vi "Fetch Measurement (Others).vi"(0 "VISA resource name":refnum<visa-resource-name>, 5 "Timeout (10000 ms)":i32=10000 format="%.0g", 7 "Fetch Option (0)":i32, 11 "error in (no error)":errorcluster) -> (4 "VISA resource name out":refnum<visa-resource-name>, 6 "Measurement Data":dbl[](array[numeric]), 15 "error out":errorcluster)   [LabVIEW 2014, in "Agilent MXA Series.lvlib"]
doc: "Returns the results of last measurement(ACP, Burst Power, Spurious Emissions, Spectrum Emission Mask) and does not initiate data acquisition.\n\n<B>Note:</B>\n\nUse this VI only with other low-level VIs. The high-level VIs automatically incorporate this functionality. This VI does not check the instrument status."
uses:
  Agilent MXA Series.lvlib
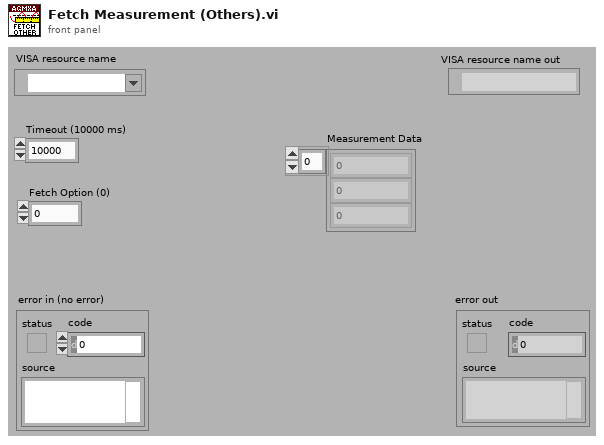
[diagram p1: front panel]
types:
  T1 = typedef "Agilent MXA Series.lvlib/Extended User Data.ctl" = cluster{"Measurement Type":i32, "Agilent MXA/EXA Model":i32}
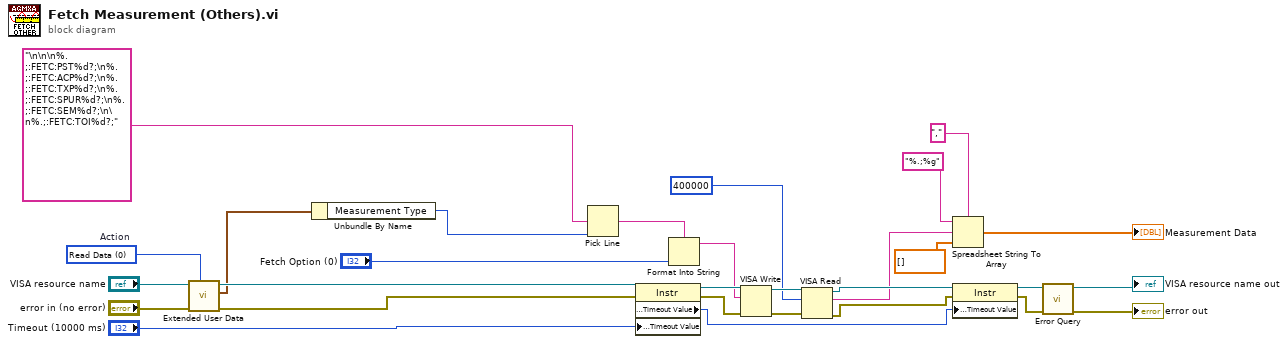
[diagram p0: block diagram]
diagram:
  w10 = 0 items=["Read Data", "Write Data", "Clear Data", "Clear ALL Data"]  # Action
  n1 = call "Extended User Data.vi"("Action (1:Write Data)"=w10, "Error In (no error)"="error in (no error)", "VISA resource name in"="VISA resource name") -> ("Error Out"=w11:errorcluster, "User Data Out"=w9:T1, "VISA resource name out"=w12:refnum<visa-resource-name>)  [unwired: 6 in]
  n2 = Unbundle By Name(w9) -> ("Measurement Type"=w8:i32)
  n3 = Pick Line(multi-line string="\n\n\n%.;:FETC:PST%d?;\n%.;:FETC:ACP%d?;\n%.;:FETC:TXP%d?;\n%.;:FETC:SPUR%d?;\n%.;:FETC:SEM%d?;\n\n%.;:FETC:TOI%d?;", line index=w8) -> (output string=w28:string)  [unwired: 1 in]
  n4 = property on="Property Node" class="Instr"(reference=w12, error in=w11, "General Settings:Timeout Value"="Timeout (10000 ms)") -> (reference out=w25:refnum<visa-resource-name>, error out=w26:errorcluster, "General Settings:Timeout Value"=w20:u32)
  n5 = Format Into String(format string=w28, "Fetch Option (0)") -> (resulting string=w1:string)  [unwired: 2 in, 1 out]
  n6 = VISA Write(VISA resource name=w25, write buffer=w1, error in (no error)=w26) -> (VISA resource name out=w23:refnum<visa-resource-name>, error out=w24:errorcluster)  [unwired: 1 out]
  n7 = VISA Read(VISA resource name=w23, byte count=400000, error in (no error)=w24) -> (VISA resource name out=w22:refnum<visa-resource-name>, read buffer=w16:string, error out=w21:errorcluster)  [unwired: 1 out]
  n8 = Spreadsheet String To Array(delimiter (Tab)=",", format string="%.;%g", spreadsheet string=w16, array type (2D Dbl)=dbl[] [] ("Measurement Data 2")) -> (array=→"Measurement Data":dbl[])
  n9 = property on="Property Node" class="Instr"(reference=w22, error in=w21, "General Settings:Timeout Value"=w20) -> (reference out=w4:refnum<visa-resource-name>, error out=w5:errorcluster)
  n10 = call "Error Query.vi"("error in (no error)"=w5, "VISA resource name"=w4) -> ("error out"=→"error out":errorcluster, "VISA resource name out"=→"VISA resource name out":refnum<visa-resource-name>)  [unwired: 6 in, 2 out]
